vi "有哪些物件呢.vi"() -> ()   [LabVIEW 2015]
panel:
  out "EveryKindOfClassNameInFront":string[][](array[string])
  out "EveryKindOfClassNameInBlock":string[][](array[string])
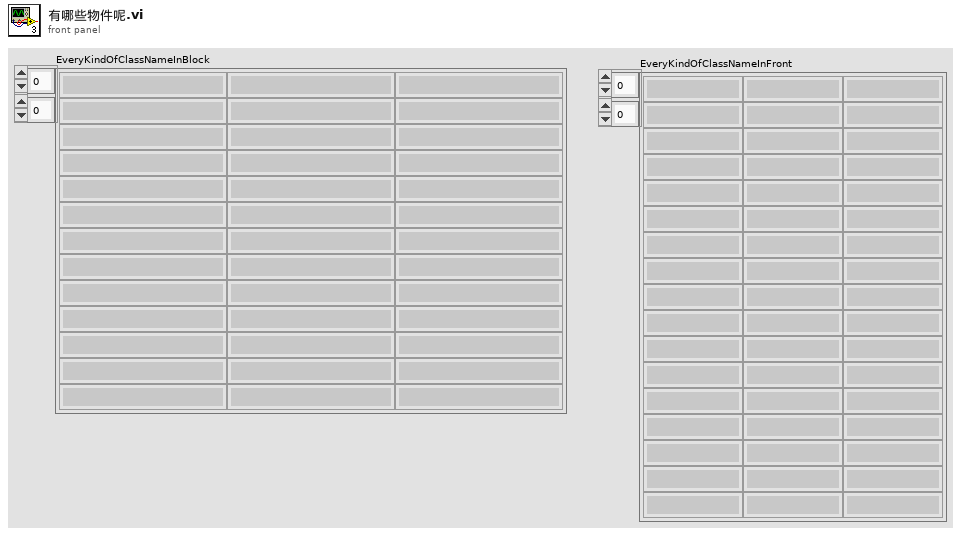
[diagram p1: front panel]
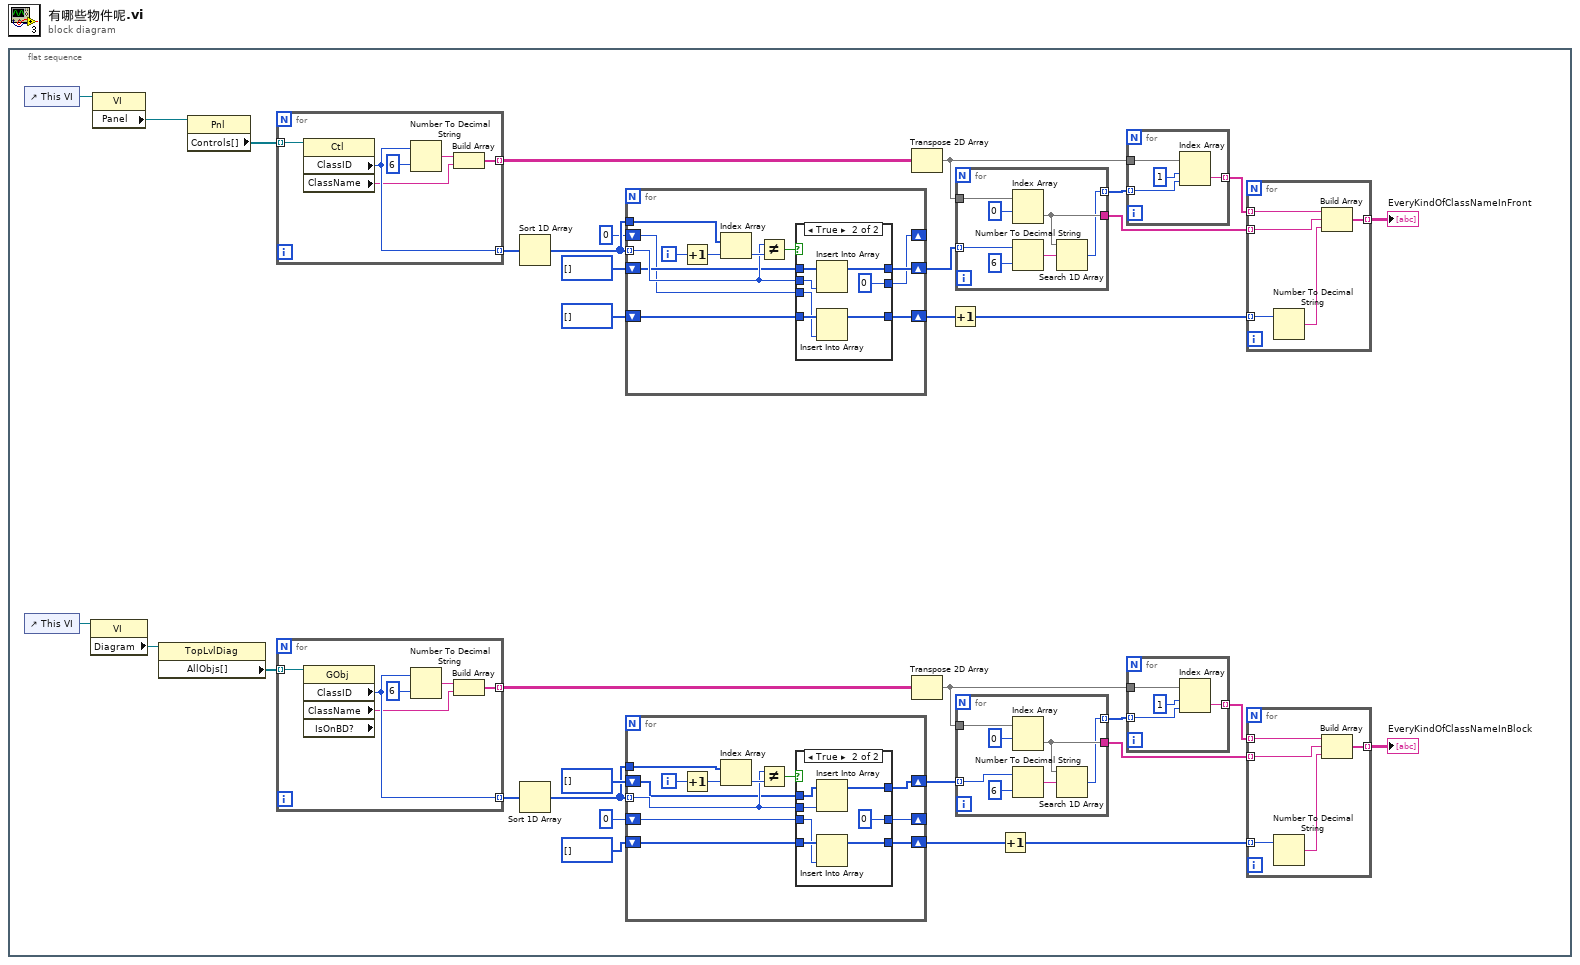
[diagram p0: block diagram]
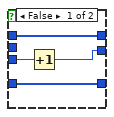
[diagram p2: hidden frame]
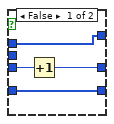
[diagram p3: hidden frame]
diagram:
  n1 = flat-sequence {
    frame #0 {
      n2 = control-ref of="This VI"() -> (w11:refnum<vi>)
      n3 = control-ref of="This VI"() -> (w32:refnum<vi>)
      n4 = property class="VI"(reference=w32) -> ("Diagram"=w33:refnum<vi>)  [unwired: 1 in, 2 out]
      n5 = property class="VI"(reference=w11) -> ("Panel"=w10:refnum<vi>)  [unwired: 1 in, 2 out]
      n6 = property class="TopLvlDiag"(reference=w33) -> ("AllObjs[]"=w18:refnum<vi>[])  [unwired: 1 in, 2 out]
      n7 = property class="Pnl"(reference=w10) -> ("Controls[]"=w12:refnum<vi>[])  [unwired: 1 in, 2 out]
      n8 = for {
        tunnel: w12 -> [w56] mode=indexing
        tunnel: [w55] -> w13 mode=indexing
        tunnel: [w52] -> w15 mode=indexing
        n9 = property class="Ctl"(reference=w56) -> ("ClassID"=w55:u32, "ClassName"=w53:string)  [unwired: 1 in, 2 out]
        n10 = Number To Decimal String(number=w55, width (-)=i16 6) -> (decimal integer string=w54:string)
        n11 = Build Array(w54, w53) -> (w52:string[])
      }
      n12 = for {
        tunnel: w18 -> [w101] mode=indexing
        tunnel: [w100] -> w31 mode=indexing
        tunnel: [w97] -> w21 mode=indexing
        n13 = property class="GObj" props=["ClassID", "ClassName", "IsOnBD?"](reference=w101) -> ("ClassID"=w100:u32, "ClassName"=w98:string)  [unwired: 1 in, 3 out]
        n14 = Number To Decimal String(number=w100, width (-)=i16 6) -> (decimal integer string=w99:string)
        n15 = Build Array(w99, w98) -> (w97:string[])
      }
      n16 = Sort 1D Array(array=w13) -> (sorted array=w9:u32[])
      n17 = Sort 1D Array(array=w31) -> (sorted array=w22:u32[])
      n18 = for {
        tunnel: w9 -> [w68]
        tunnel: w9 -> [w63] mode=indexing
        shift-right: [w61] -> w14
        shift-left: u32[] [] -> [w62]
        shift-right: [w59] -> w2
        shift-left: u32[] [] -> [w60]
        shift-right: [w57] -> _
        shift-left: 0 -> [w58]
        i -> [w67]
        n19 = Increment(x=w67) -> (x+1=w66:i32)
        n20 = Index Array(array=w68, index=w66) -> (element=w65:u32)
        n21 = Not Equal?(x=w63, y=w65) -> (x != y?=w64:bool)
        n22 = case shown="True" w64 {
          tunnel: w62 -> [w72 w78]
          tunnel: [w72 w79] -> w61
          tunnel: w63 -> [_ w77]
          tunnel: w60 -> [w69 w76]
          tunnel: [w69 w75] -> w59
          tunnel: w58 -> [w71 w74]
          tunnel: [w70 0] -> w57
          frame False {
            n23 = Increment(x=w71) -> (x+1=w70:i32)
          }
          frame True {
            n24 = Insert Into Array(array=w78, new element=w77) -> (w79:u32[])  [unwired: 1 in]
            n25 = Insert Into Array(array=w76, new element=w74) -> (w75:u32[])  [unwired: 1 in]
          }
        }
      }
      n26 = for {
        tunnel: w22 -> [w113]
        tunnel: w22 -> [w110] mode=indexing
        shift-right: [w108] -> w23
        shift-left: u32[] [] -> [w109]
        shift-right: [w106] -> _
        shift-left: 0 -> [w107]
        shift-right: [w104] -> w20
        shift-left: u32[] [] -> [w105]
        i -> [w103]
        n27 = Increment(x=w103) -> (x+1=w102:i32)
        n28 = Index Array(array=w113, index=w102) -> (element=w112:u32)
        n29 = Not Equal?(x=w110, y=w112) -> (x != y?=w111:bool)
        n30 = case shown="True" w111 {
          tunnel: w109 -> [w117 w123]
          tunnel: [w117 w124] -> w108
          tunnel: w110 -> [_ w122]
          tunnel: w107 -> [w116 w119]
          tunnel: [w115 0] -> w106
          tunnel: w105 -> [w114 w121]
          tunnel: [w114 w120] -> w104
          frame False {
            n31 = Increment(x=w116) -> (x+1=w115:i32)
          }
          frame True {
            n32 = Insert Into Array(array=w123, new element=w122) -> (w124:u32[])  [unwired: 1 in]
            n33 = Insert Into Array(array=w121, new element=w119) -> (w120:u32[])  [unwired: 1 in]
          }
        }
      }
      n34 = Transpose 2D Array(2D array=w15) -> (transposed array=w17:string[][])
      n35 = Transpose 2D Array(2D array=w21) -> (transposed array=w29:string[][])
      n36 = Increment(x=w2) -> (x+1=w1:u32[])
      n37 = for {
        tunnel: w14 -> [w47] mode=indexing
        tunnel: w17 -> [w49]
        tunnel: [w48] -> w6
        tunnel: [w44] -> w16 mode=indexing
        n38 = Index Array(array=w49, index (row)=0) -> (element=w48:string[])  [unwired: 1 in]
        n39 = Number To Decimal String(number=w47, width (-)=i16 6) -> (decimal integer string=w46:string)
        n40 = Search 1D Array(1D array=w48, element=w46) -> (index of element=w44:i32)  [unwired: 1 in]
      }
      n41 = for {
        tunnel: w23 -> [w92] mode=indexing
        tunnel: w29 -> [w94]
        tunnel: [w93] -> w27
        tunnel: [w89] -> w30 mode=indexing
        n42 = Index Array(array=w94, index (row)=0) -> (element=w93:string[])  [unwired: 1 in]
        n43 = Number To Decimal String(number=w92, width (-)=i16 6) -> (decimal integer string=w91:string)
        n44 = Search 1D Array(1D array=w93, element=w91) -> (index of element=w89:i32)  [unwired: 1 in]
      }
      n45 = Increment(x=w20) -> (x+1=w19:u32[])
      n46 = for {
        tunnel: w16 -> [w41] mode=indexing
        tunnel: w17 -> [w43]
        tunnel: [w40] -> w7 mode=indexing
        n47 = Index Array(array=w43, index (row)=1, index (col)=w41) -> (element=w40:string)
      }
      n48 = for {
        tunnel: w30 -> [w86] mode=indexing
        tunnel: w29 -> [w88]
        tunnel: [w85] -> w28 mode=indexing
        n49 = Index Array(array=w88, index (row)=1, index (col)=w86) -> (element=w85:string)
      }
      n50 = for {
        tunnel: w7 -> [w39] mode=indexing
        tunnel: w6 -> [w38] mode=indexing
        tunnel: [w37] -> w5 mode=indexing
        tunnel: w1 -> [w36] mode=indexing
        n51 = Number To Decimal String(number=w36) -> (decimal integer string=w35:string)  [unwired: 1 in]
        n52 = Build Array(w39, w38, w35) -> (w37:string[])
      }
      "EveryKindOfClassNameInFront" <- w5
      n53 = for {
        tunnel: w28 -> [w84] mode=indexing
        tunnel: w27 -> [w83] mode=indexing
        tunnel: [w82] -> w26 mode=indexing
        tunnel: w19 -> [w81] mode=indexing
        n54 = Number To Decimal String(number=w81) -> (decimal integer string=w80:string)  [unwired: 1 in]
        n55 = Build Array(w84, w83, w80) -> (w82:string[])
      }
      "EveryKindOfClassNameInBlock" <- w26
    }
  }
